vi "Auto Path Names.vi"() -> (3 "Path Names":string[](array[string]))   [LabVIEW 2019]
uses:
  <vilib>/Rock Robotics/Network Tables/NT Read String.vi
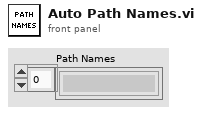
[diagram p1: front panel]
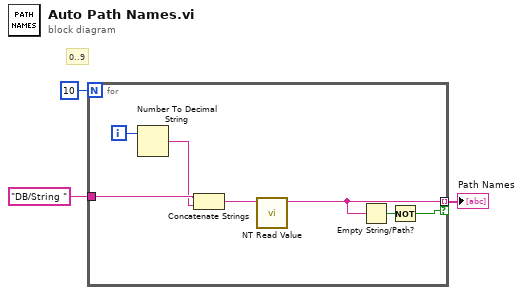
[diagram p0: block diagram]
diagram:
  # "0..9"
  n1 = for {
    N: 10 -> [_]
    tunnel: "DB/String " -> [w10]
    tunnel: [w7] -> w1 mode=indexing if=w5
    i -> [w4]
    n2 = Number To Decimal String(number=w4) -> (decimal integer string=w9:string)  [unwired: 1 in]
    n3 = Concatenate Strings(w10, w9) -> (w8:string)
    n4 = call-poly <vilib>:"NT Read Value.vi"("Name"=w8) -> ("String"=w7:string)  [unwired: 9 in, 1 out]
    n5 = Empty String/Path?(string/path=w7) -> (empty?=w6:bool)
    n6 = Not(x=w6) -> (.not. x?=w5:bool)
  }
  "Path Names" <- w1
